vi "Initialize PJVS.vi"(7 "Abort Refnum":refnum<vi>, 8 "error in (no error)":errorcluster, 11 "PJVS setup":T1={"PJVS type"=enum."AC-supraVOLTcontrol", "Status Refnum"=refnum, "AC-supraVOLTcontrol"={"IP address:port (0.0.0.0:0000)"="0.0.0.0:0000", "Timeouts"={"TCP Read & Write (ms)"=7000, "Sensors readout"=5000, "PJVS setup"=10000, "Nullmeter readout"=5000, "Multiplexer setup"=3000, "57XX setup"=15000, "Generator setup"=5000, "Synthesizer setup"=3000, "Sampler readout"=10000}, "Simulation mode"=FALSE, "Debug mode"=FALSE}, "NPL bias source"={"DataSocketCluster"={"Server Machine"="CZC", "Client Machine"="localhost", "Data"="P2", "TimeStamp"=0.0, "Count"=1, "Target Process"="General Server"}}, "Manual PJVS"={"PJVS frequency (Hz)"=0.0, "Reference voltages (V)"=[], "File with PJVS voltages"=path ""}, "VTT PJVS"={"some VTT only property"=""}} {"NPL bias source"."DataSocketCluster"."TimeStamp" format="%.2f"}) -> (0 "error out":errorcluster, 3 "PJVS setup out":T1={"PJVS type"=enum."AC-supraVOLTcontrol", "Status Refnum"=refnum, "AC-supraVOLTcontrol"={"IP address:port (0.0.0.0:0000)"="0.0.0.0:0000", "Timeouts"={"TCP Read & Write (ms)"=7000, "Sensors readout"=5000, "PJVS setup"=10000, "Nullmeter readout"=5000, "Multiplexer setup"=3000, "57XX setup"=15000, "Generator setup"=5000, "Synthesizer setup"=3000, "Sampler readout"=10000}, "Simulation mode"=FALSE, "Debug mode"=FALSE}, "NPL bias source"={"DataSocketCluster"={"Server Machine"="CZC", "Client Machine"="localhost", "Data"="P2", "TimeStamp"=0.0, "Count"=1, "Target Process"="General Server"}}, "Manual PJVS"={"PJVS frequency (Hz)"=0.0, "Reference voltages (V)"=[], "File with PJVS voltages"=path ""}, "VTT PJVS"={"some VTT only property"=""}} {"NPL bias source"."DataSocketCluster"."TimeStamp" format="%.2f"})   [LabVIEW 2020]
doc: "Initialize the PJVS. Calls the initialization routine of the actual driver."
uses:
  Type definitions/PJVS.ctl
  Type definitions/PJVS Type.ctl
  external libraries/acsvcontrol-driver/Public/Type Definitions/Timeouts.ctl
  external libraries/JV modified NPL Bias source/DataSocketCluster external.ctl
  external libraries/acsvcontrol-driver/Public/Type Definitions/Debug status.ctl
  external libraries/acsvcontrol-driver/ACSVcontrol-driver.lvlib
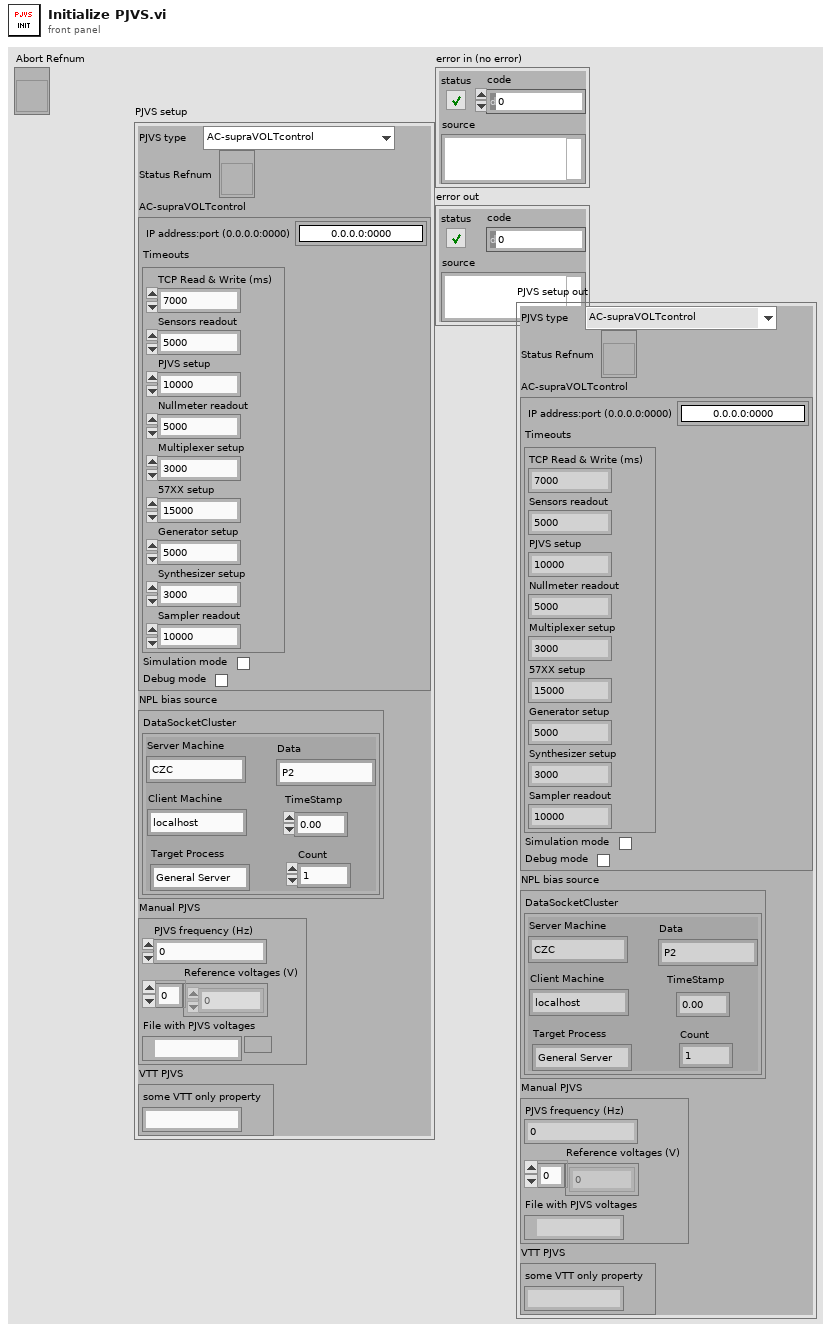
[diagram p1: front panel]
types:
  T1 = typedef "PJVS.ctl" = cluster{"PJVS type":T2, "Status Refnum":refnum<vi>, "AC-supraVOLTcontrol":cluster{"IP address:port (0.0.0.0:0000)":string, "Timeouts":T3, "Simulation mode":bool, "Debug mode":bool}, "NPL bias source":cluster{"DataSocketCluster":T4}, "Manual PJVS":cluster{"PJVS frequency (Hz)":dbl, "Reference voltages (V)":dbl[], "File with PJVS voltages":path}, "VTT PJVS":cluster{"some VTT only property":string}}
  T2 = typedef "PJVS Type.ctl" = enum16{"AC-supraVOLTcontrol", "JV modified NPL bias control", "Manual PJVS", "VTT PJVS"}
  T3 = typedef "ACSVcontrol-driver.lvlib/Timeouts.ctl" = cluster{"TCP Read & Write (ms)":i32, "Sensors readout":i32, "PJVS setup":i32, "Nullmeter readout":i32, "Multiplexer setup":i32, "57XX setup":i32, "Generator setup":i32, "Synthesizer setup":i32, "Sampler readout":i32}
  T4 = typedef "DataSocketCluster external.ctl" = cluster{"Server Machine":string, "Client Machine":string, "Data":string, "TimeStamp":dbl, "Count":i32, "Target Process":string}
  T5 = typedef "ACSVcontrol-driver.lvlib/Debug status.ctl" = enum16{"No change", "Off", "On"}
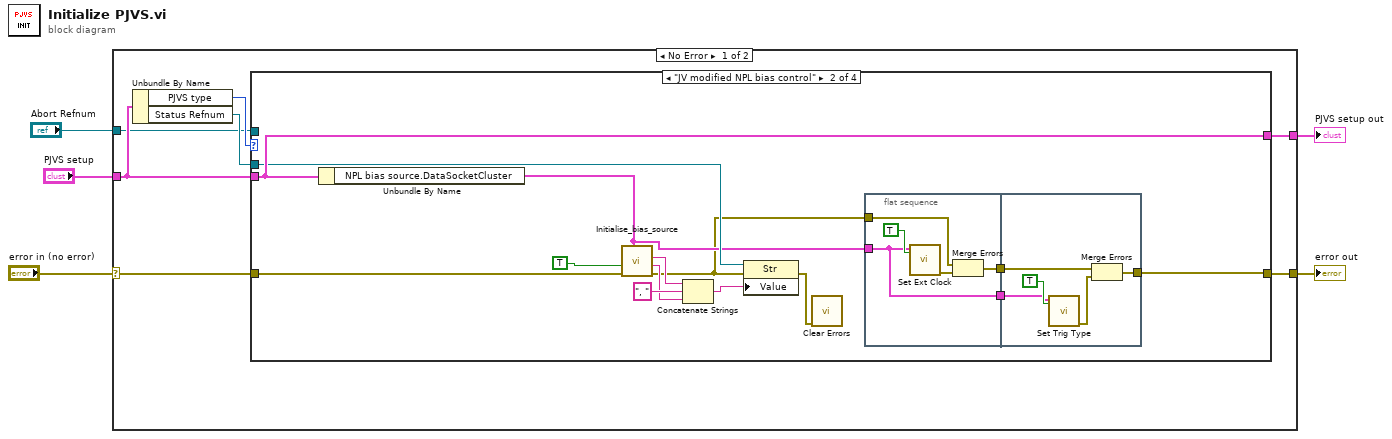
[diagram p0: block diagram]
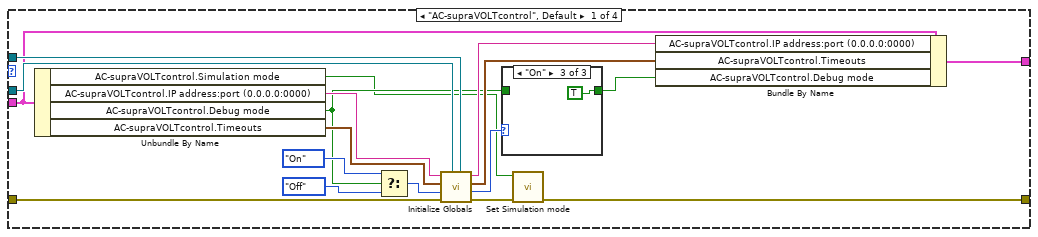
[diagram p2: hidden frame]
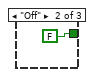
[diagram p4: hidden frame]
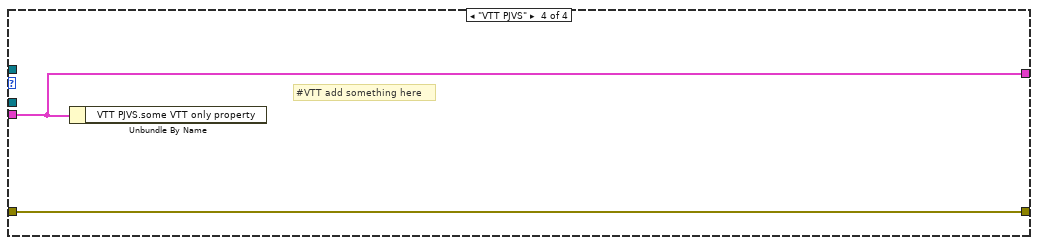
[diagram p6: hidden frame]
diagram:
  n1 = case shown="No Error" "error in (no error)" {
    selector: "error in (no error)" -> [w8 w63]
    tunnel: "PJVS setup" -> [w11 w62]
    tunnel: [w9 w63] -> w4
    tunnel: [w7 w62] -> w2
    tunnel: "Abort Refnum" -> [w6 _]
    frame No Error {
      n2 = Unbundle By Name(w11) -> ("PJVS type"=w12:T2, "Status Refnum"=w10:refnum<vi>)
      n3 = case shown="\"JV modified NPL bias control\"" w12 {
        tunnel: w11 -> [w25 w47 w59 w61]
        tunnel: w10 -> [w29 w40 _ _]
        tunnel: w6 -> [w28 _ _ _]
        tunnel: w8 -> [w26 w45 w58 w60]
        tunnel: [w14 w38 w58 w60] -> w9
        tunnel: [w22 w47 w59 w61] -> w7
        frame "AC-supraVOLTcontrol", Default {
          n4 = Unbundle By Name(w25) -> ("AC-supraVOLTcontrol.Simulation mode"=w13:bool, "AC-supraVOLTcontrol.IP address:port (0.0.0.0:0000)"=w30:string, "AC-supraVOLTcontrol.Debug mode"=w16:bool, "AC-supraVOLTcontrol.Timeouts"=w27:T3)
          n5 = Select(t=Debug_status."On" ("Debug mode"), s=w16, f=Debug_status."Off" ("Debug mode")) -> (s? t:f=w19:T5)
          n6 = call "Initialize Globals.vi"("Abort Refnum"=w28, "Status Refnum"=w29, "error in (pass through)"=w26, "Debug mode"=w19, "Timeouts"=w27, "IP address:port (0.0.0.0:0000)"=w30) -> ("error out"=w15:errorcluster, "Debug mode out"=w18:T5, "Timeouts out"=w23:T3, "IP address:port out"=w24:string)  [unwired: 2 out]
          n7 = case shown="\"On\"" w18 {
            tunnel: [w31 FALSE ("AC-supraVOLTcontrol.Debug mode") TRUE ("AC-supraVOLTcontrol.Debug mode")] -> w17
            tunnel: w16 -> [w31 _ _]
            frame "No change", Default {
            }
            frame "Off" {
            }
            frame "On" {
            }
          }
          n8 = call "Set Simulation mode.vi"("error in (no error)"=w15, "Simulation mode (T)"=w13) -> ("error out (passthrough)"=w14:errorcluster)  [unwired: 9 in]
          n9 = Bundle By Name(cluster=w25, "AC-supraVOLTcontrol.IP address:port (0.0.0.0:0000)"=w24, "AC-supraVOLTcontrol.Timeouts"=w23, "AC-supraVOLTcontrol.Debug mode"=w17) -> (w22:T1)
        }
        frame "JV modified NPL bias control" {
          n10 = Unbundle By Name(w47) -> ("NPL bias source.DataSocketCluster"=w37:T4)
          n11 = call "Initialise_bias_source.vi"("output cluster"=w37, "error in (no error)"=w45, "Load bias parameters"=TRUE) -> ("error out"=w35:errorcluster, "Response to Load bias parameters"=w42:string, "Response Initialise"=w43:string)  [unwired: 6 in]
          n12 = Concatenate Strings(w43, ", " ("string"), w42) -> (w41:string)
          n13 = property class="Str"(reference=w40, error in=w35, "Value"=w41) -> (error out=w34:errorcluster)  [unwired: 1 out]
          n14 = call <vilib>:"Clear Errors.vi"("error in (no error)"=w34) -> ()  [unwired: 5 in, 2 out]
          n15 = flat-sequence {
            tunnel: [w50] -> w39
            tunnel: w35 -> [w52]
            tunnel: w37 -> [w48]
            tunnel: [w48] -> w36
            tunnel: [w55] -> w38
            tunnel: w39 -> [w57]
            tunnel: w36 -> [w53]
            frame #0 {
              n16 = call "Set Ext Clock.vi"("Requested state of Ext clock"=TRUE, "machine"=w48) -> ("error out"=w51:errorcluster)  [unwired: 8 in, 1 out]
              n17 = Merge Errors(w52, w51) -> (w50:errorcluster)
            }
            frame #1 {
              n18 = call "Set Trig Type.vi"("Requested state of Trig (off: Update)"=TRUE, "machine"=w53) -> ("error out"=w56:errorcluster)  [unwired: 8 in, 1 out]
              n19 = Merge Errors(w57, w56) -> (w55:errorcluster)
            }
          }
        }
        frame "Manual PJVS" {
          # "Nothing to do for manually set PJVS"
        }
        frame "VTT PJVS" {
          # "#VTT add something here"
          n20 = Unbundle By Name(w61) -> ()  [unwired: 1 out]
        }
      }
    }
    frame Error {
    }
  }
  "error out" <- w4
  "PJVS setup out" <- w2
